vi "MFCInit.vi"() -> (0 "MFC error out":errorcluster, 3 "MFC VISA out":refnum<visa-resource-name>)   [LabVIEW 2018]
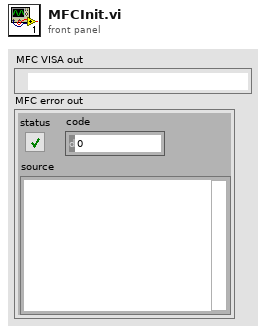
[diagram p1: front panel]
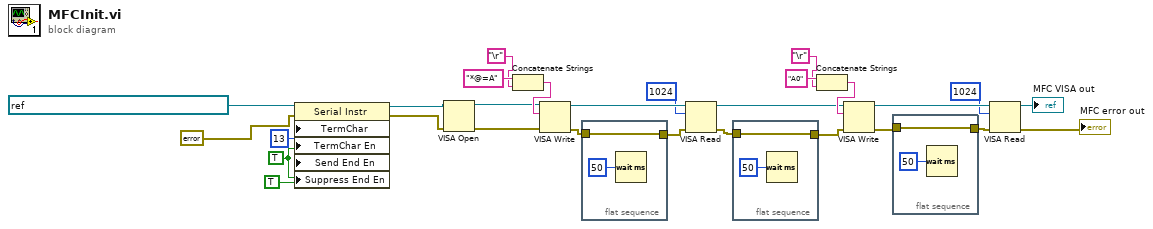
[diagram p0: block diagram]
diagram:
  w7 = TRUE ("Message Based Settings:Termination Character Enable")
  n1 = property class="Serial Instr"(reference=refnum<visa-resource-name> "TCPIP0::192.168.2.110::4002::SOCKET" ("VISA resource name"), error in=errorcluster {"status"=FALSE, "code"=0, "source"=""} ("error in (no error)"), "TermChar"=u8 13 ("Message Based Settings:Termination Character"), "TermChar En"=w7, "Send End En"=TRUE ("Message Based Settings:Send End Enable"), "Suppress End En"=w7) -> (reference out=w3:refnum<visa-resource-name>, error out=w4:errorcluster)
  n2 = VISA Open(error in (no error)=w4, VISA resource name=w3) -> (VISA resource name=w1:refnum<visa-resource-name>, error out=w2:errorcluster)  [unwired: 3 in]
  n3 = Concatenate Strings("*@=A" ("write buffer"), "\r") -> (w27:string)
  n4 = VISA Write(VISA resource name=w1, write buffer=w27, error in (no error)=w2) -> (VISA resource name out=w25:refnum<visa-resource-name>, error out=w18:errorcluster)  [unwired: 1 out]
  n5 = flat-sequence {
    tunnel: w18 -> [w30]
    tunnel: [w30] -> w17
    frame #0 {
      n6 = Wait (ms)(milliseconds to wait=u32 50) -> ()  [unwired: 1 out]
    }
  }
  n7 = VISA Read(VISA resource name=w25, byte count=u32 1024, error in (no error)=w17) -> (VISA resource name out=w14:refnum<visa-resource-name>, error out=w16:errorcluster)  [unwired: 2 out]
  n8 = flat-sequence {
    tunnel: w16 -> [w32]
    tunnel: [w32] -> w15
    frame #0 {
      n9 = Wait (ms)(milliseconds to wait=u32 50) -> ()  [unwired: 1 out]
    }
  }
  n10 = Concatenate Strings("A0" ("write buffer"), "\r") -> (w22:string)
  n11 = VISA Write(VISA resource name=w14, write buffer=w22, error in (no error)=w15) -> (VISA resource name out=w20:refnum<visa-resource-name>, error out=w13:errorcluster)  [unwired: 1 out]
  n12 = flat-sequence {
    tunnel: w13 -> [w34]
    tunnel: [w34] -> w12
    frame #0 {
      n13 = Wait (ms)(milliseconds to wait=u32 50) -> ()  [unwired: 1 out]
    }
  }
  n14 = VISA Read(VISA resource name=w20, byte count=u32 1024, error in (no error)=w12) -> (VISA resource name out=→"MFC VISA out":refnum<visa-resource-name>, error out=→"MFC error out":errorcluster)  [unwired: 2 out]
